vi "Get Data.vi"(8 "error in":errorcluster, 11 "CPC in":refnum<class "CPC.lvclass">) -> (0 "error out":errorcluster, 2 "Data Out":refnum<class "CPC Data.lvclass">, 3 "CPC out":refnum<class "CPC.lvclass">)   [LabVIEW 2013, in "CPC.lvclass"]
uses:
  CPC.lvclass
  Data/CPC Data.lvclass
  Data/CPC Data.lvclass/CPC Data.ctl
  Data/Write Buffer Counts.vi
  Read 1s Buffer.vi
  Read Front Panel Concentration.vi
  Read Condenser Temperature.vi
  Read Saturator Temperature.vi
  Read Environment.vi
  Reusable/Data/Write measTime.vi
  Data/Write FP [N].vi
  Data/Write instrT.vi
  Data/Write sysReady.vi
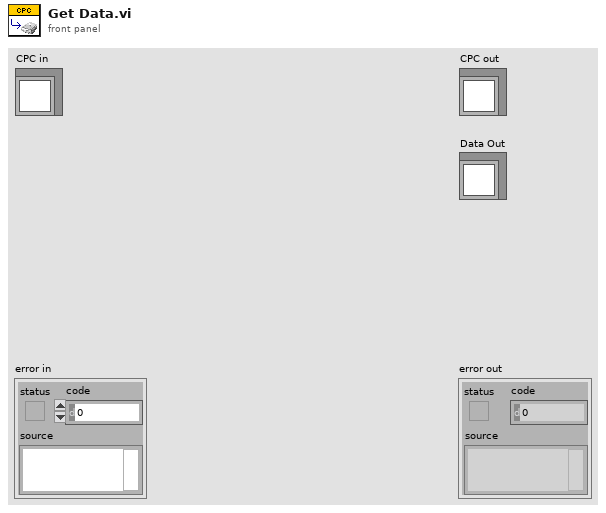
[diagram p1: front panel]
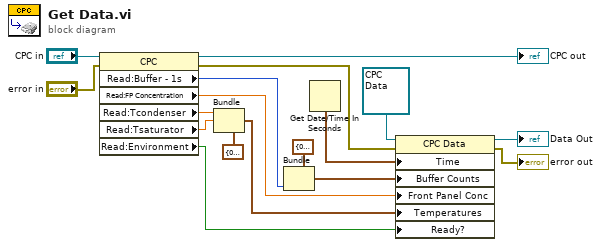
[diagram p0: block diagram]
diagram:
  n1 = property class="CPC"(reference="CPC in", error in="error in") -> (reference out=→"CPC out":refnum<class "CPC.lvclass">, error out=w12:errorcluster, "Read:Buffer - 1s"=w9:i32, "Read:FP Concentration"=w11:dbl, "Read:Tcondenser"=w6:dbl, "Read:Tsaturator"=w5:dbl, "Read:Environment"=w3:bool)
  n2 = Bundle(cluster=cluster{"cond T":dbl, "sat T":dbl, "opt T":dbl} {"cond T"=0.0, "sat T"=0.0, "opt T"=0.0} ("Temperatures"), "cond T"=w6, "sat T"=w5) -> (w4:cluster{"cond T":dbl, "sat T":dbl, "opt T":dbl})  [unwired: 1 in]
  n3 = Bundle(cluster=cluster{"200 s":u32, "20 s":u32, "1 s":u32} {"200 s"=0, "20 s"=0, "1 s"=0} ("Buffer Counts"), "1 s"=w9) -> (w8:cluster{"200 s":u32, "20 s":u32, "1 s":u32})  [unwired: 2 in]
  n4 = Get Date/Time In Seconds() -> (seconds since 1Jan1904=w13:timestamp)
  n5 = property class="CPC Data"(reference=refnum<class "CPC Data.lvclass"> refnum ("CPC Data"), error in=w12, "Time"=w13, "Buffer Counts"=w8, "Front Panel Conc"=w11, "Temperatures"=w4, "Ready?"=w3) -> (reference out=→"Data Out":refnum<class "CPC Data.lvclass">, error out=→"error out":errorcluster)
